vi "Write Response to Stream.vi"(7 "Close? (T)":bool=TRUE, 8 "error in (no error)":errorcluster, 9 "Stream in":refnum<k5>, 11 "Response in":refnum<class "Response.lvclass">) -> (0 "error out":errorcluster, 3 "Response out":refnum<class "Response.lvclass">)   [LabVIEW 2020, in "HTTP Utils.lvlib" / "Response.lvclass"]
uses:
  Response.lvclass
  lv-stream/stream/Stream/Stream.lvclass/Stream.ctl
  lv-stream/stream/Stream/Dispatch Sniffer Data.vi
  lv-stream/stream/Stream/Prepared.vi
  lv-stream/stream/Endpoint/Cast Sniffer Callback.vi
  lv-stream/stream/Error Bad State.vi
  <vilib>/Utility/error.llb/Error Cluster From Error Code.vi
  lv-stream/stream/Stream/Stream.lvclass
  Response.lvclass/Response.ctl
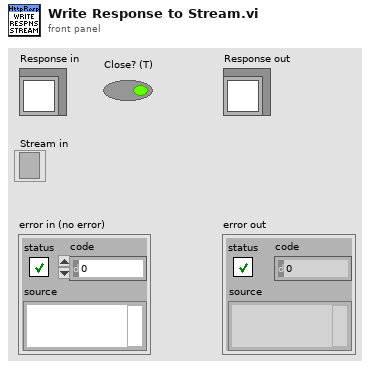
[diagram p1: front panel]
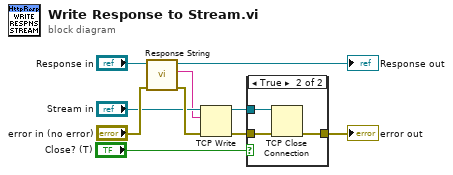
[diagram p0: block diagram]
diagram:
  n1 = call-dynamic "Response String.vi"("error in (no error)"="error in (no error)", "Response in"="Response in") -> ("error out"=w3:errorcluster, "Response String"=w1:string, "Response out"=→"Response out":refnum<class "Response.lvclass">)  [unwired: 7 in]
  n2 = TCP Write(connection ID="Stream in", data in=w1, error in (no error)=w3) -> (connection ID out=w5:refnum<k5>, error out=w4:errorcluster)  [unwired: 1 in, 1 out]
  n3 = case shown="True" "Close? (T)" {
    tunnel: w4 -> [w11 w13]
    tunnel: w5 -> [_ w14]
    tunnel: [w11 w12] -> w7
    frame False {
    }
    frame True {
      n4 = TCP Close Connection(connection ID=w14, error in (no error)=w13) -> (error out=w12:errorcluster)  [unwired: 1 in, 1 out]
    }
  }
  "error out" <- w7
